vi "Calculate Serial Number.vi"(8 "error in (no error)":errorcluster, 11 "Vendor ID (AA)":string="AA") -> (0 "error out":errorcluster, 3 "UUT Serial  No.":string="AA48234912")   [LabVIEW 2013]
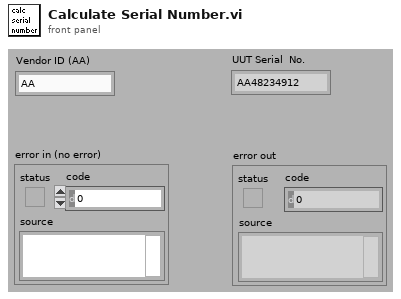
[diagram p1: front panel]
types:
  T1 = typedef "LVDateTimeRec.ctl" = cluster{"fractional second":dbl, "second":i32, "minute":i32, "hour":i32, "day of month":i32, "month":i32, "year":i32, "day of week":i32, "day of year":i32, "DST":i32}
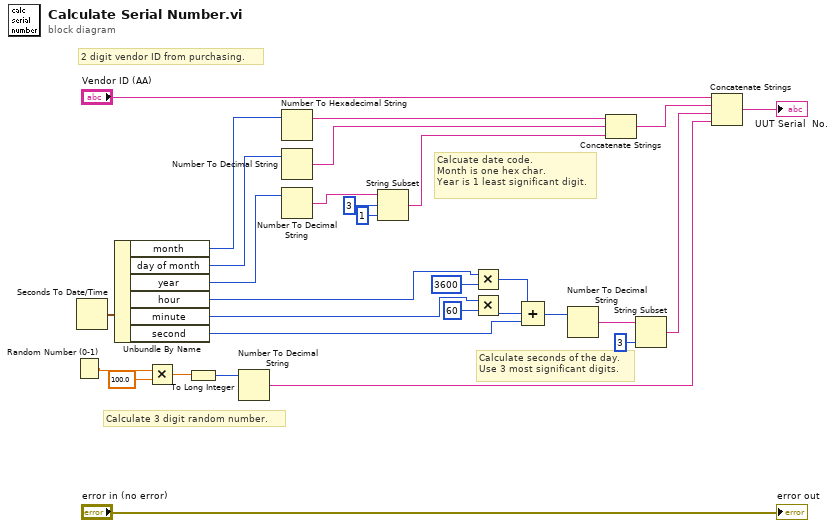
[diagram p0: block diagram]
diagram:
  # "2 digit vendor ID from purchasing."
  # "Calculate 3 digit random number."
  # "Calculate seconds of the day.\nUse 3 most significant digits."
  # "Calcuate date code.\nMonth is one hex char.\nYear is 1 least significant digit."
  n1 = Random Number (0-1)() -> (number: 0 to 1=w29:dbl)
  n2 = Seconds To Date/Time() -> (date time rec=w22:T1)  [unwired: 2 in]
  n3 = Unbundle By Name(w22) -> ("month"=w10:i32, "day of month"=w9:i32, "year"=w8:i32, "hour"=w21:i32, "minute"=w18:i32, "second"=w15:i32)
  n4 = Multiply(x=w29, y=100.0) -> (x*y=w27:dbl)
  n5 = To Long Integer(number=w27) -> (32bit integer=w26:i32)
  n6 = Number To Decimal String(number=w26) -> (decimal integer string=w25:string)  [unwired: 1 in]
  n7 = Number To Hexadecimal String(2:w10) -> (0:w3:string)  [unwired: 1 in]
  n8 = Number To Decimal String(number=w9) -> (decimal integer string=w2:string)  [unwired: 1 in]
  n9 = Number To Decimal String(number=w8) -> (decimal integer string=w4:string)  [unwired: 1 in]
  n10 = String Subset(string=w4, offset (0)=3, length (rest)=1 ("length (rest)")) -> (substring=w1:string)
  n11 = Multiply(x=w21, y=3600) -> (x*y=w17:i32)
  n12 = Multiply(x=w18, y=60) -> (x*y=w16:i32)
  n13 = Compound Arithmetic op=ADD(w17, w16, w15) -> (w14:i32)
  n14 = Number To Decimal String(number=w14) -> (decimal integer string=w13:string)  [unwired: 1 in]
  n15 = Concatenate Strings(w3, w2, w1) -> (w6:string)
  n16 = String Subset(string=w13, length (rest)=3 ("length (rest)")) -> (substring=w11:string)  [unwired: 1 in]
  n17 = Concatenate Strings("Vendor ID (AA)", w6, w11, w25) -> (→"UUT Serial  No.":string)
  "error out" <- "error in (no error)"
